vi "fgv_stop_local.vi"(7 "cmd":T1, 10 "error in (no error)":errorcluster) -> (2 "error out":errorcluster, 3 "stop":bool)   [LabVIEW 2019]
uses:
  _ctrl/init-r-stop.ctl
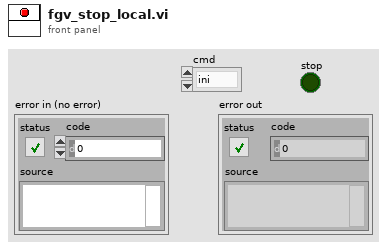
[diagram p1: front panel]
types:
  T1 = typedef "init-r-stop.ctl" = enum16{"ini", "read", "stop"}
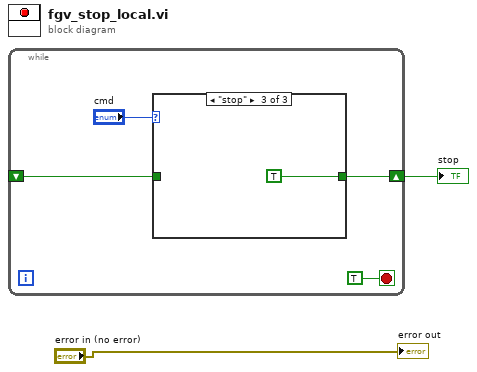
[diagram p0: block diagram]
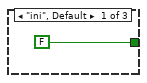
[diagram p2: hidden frame]
diagram:
  n1 = while {
    shift-right: [w4] -> w2
    shift-left: _ -> [w3]
    stop <- TRUE stop-if-true
    n2 = case shown="\"stop\"" "cmd" {
      tunnel: [FALSE w8 TRUE] -> w4
      tunnel: w3 -> [_ w8 _]
      frame "ini", Default {
      }
      frame "read" {
      }
      frame "stop" {
      }
    }
  }
  "stop" <- w2
  "error out" <- "error in (no error)"
